vi "Get Page VI.vi"(8 "error in (no error)":errorcluster, 9 "GUID":string, 10 "Item Ref":T1 format="%.0x", 11 "System Explorer Dispatcher Implementation in":refnum<class "System Explorer Dispatcher Implementation.lvclass">) -> (0 "error out":errorcluster, 2 "page reference":refnum<vi>, 3 "System Explorer Dispatcher Implementation out":refnum<class "System Explorer Dispatcher Implementation.lvclass">)   [LabVIEW 2020, in "Communication Bus Template System Explorer.lvlib" / "Implementation.lvlib" / "System Explorer Dispatcher Implementation.lvclass"]
uses:
  System Explorer Dispatcher Implementation.lvclass
  <vilib>/NI VeriStand/Custom Device API/Custom Device Item Ref.ctl
  Scripting/Constants.vi
  System Explorer/Implementation.lvlib
  Scripting/Communication Bus Template Scripting.lvlib
  <vilib>/NI VeriStand/Custom Device API/Custom Device API.lvlib
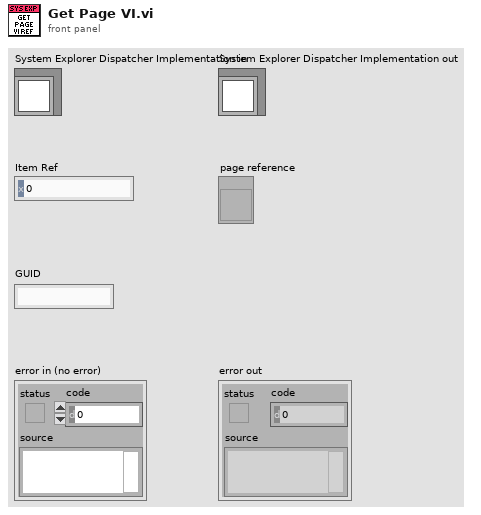
[diagram p1: front panel]
types:
  T1 = typedef "Custom Device API.lvlib/Custom Device Item Ref.ctl" = u64
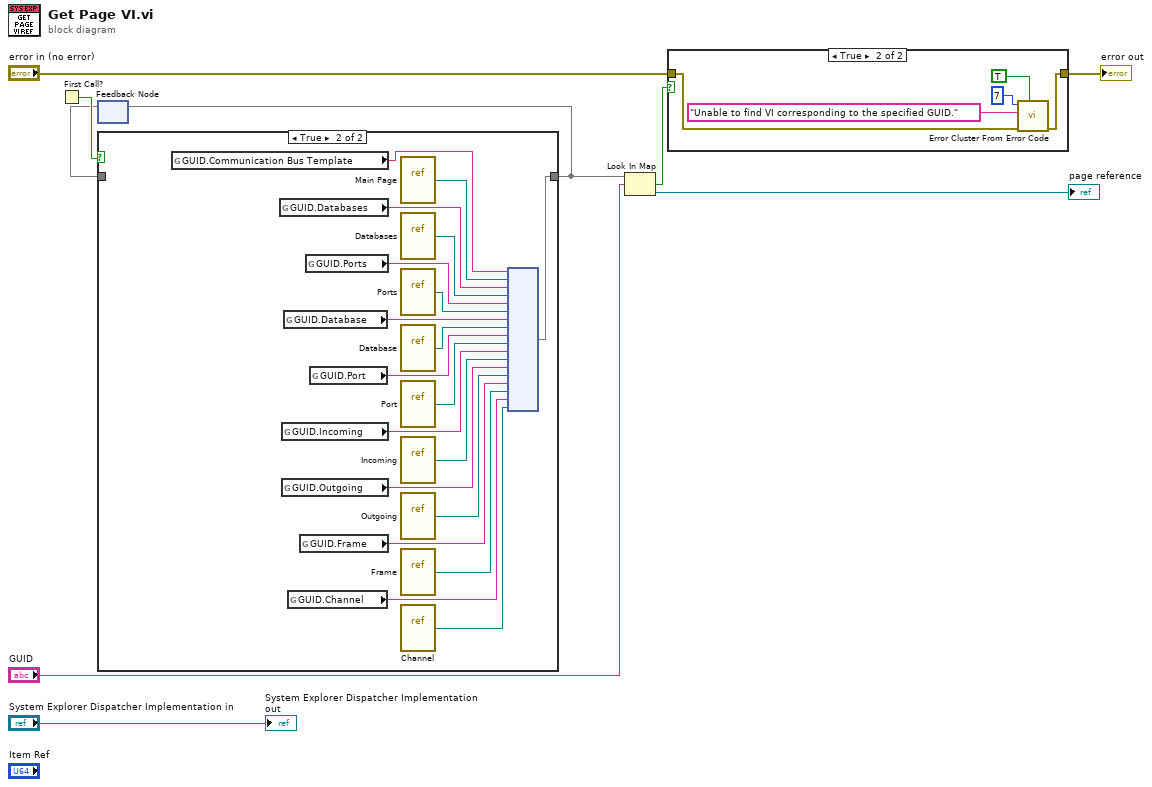
[diagram p0: block diagram]
diagram:
  n1 = First Call?() -> (First Call?: T/F=w8:bool)
  n2 = feedback #1() -> (w7:map{string, refnum<vi>})  [unwired: 1 in]
  n3 = case shown="True" w8 {
    tunnel: [w10 w29] -> w6
    tunnel: w7 -> [w10 _]
    frame False {
    }
    frame True {
      n4 = global read "Constants.vi" "GUID.Communication Bus Template"() -> (w27:string)
      n5 = global read "Constants.vi" "GUID.Databases"() -> (w25:string)
      n6 = global read "Constants.vi" "GUID.Incoming"() -> (w18:string)
      n7 = global read "Constants.vi" "GUID.Outgoing"() -> (w16:string)
      n8 = global read "Constants.vi" "GUID.Database"() -> (w22:string)
      n9 = global read "Constants.vi" "GUID.Channel"() -> (w11:string)
      n10 = global read "Constants.vi" "GUID.Frame"() -> (w14:string)
      n11 = global read "Constants.vi" "GUID.Ports"() -> (w24:string)
      n12 = global read "Constants.vi" "GUID.Port"() -> (w20:string)
      n13 = vi-ref "Main Page.vi"() -> (w28:refnum<vi>)
      n14 = vi-ref "Databases.vi"() -> (w26:refnum<vi>)
      n15 = vi-ref "Ports.vi"() -> (w23:refnum<vi>)
      n16 = vi-ref "Database.vi"() -> (w21:refnum<vi>)
      n17 = vi-ref "Port.vi"() -> (w19:refnum<vi>)
      n18 = vi-ref "Incoming.vi"() -> (w17:refnum<vi>)
      n19 = vi-ref "Outgoing.vi"() -> (w15:refnum<vi>)
      n20 = vi-ref "Frame.vi"() -> (w13:refnum<vi>)
      n21 = vi-ref "Channel.vi"() -> (w12:refnum<vi>)
      n22 = node(w27, w28, w25, w26, w24, w23, w22, w21, w20, w19, w18, w17, w16, w15, w14, w13, w11, w12) -> (w29:map{string, refnum<vi>})
    }
  }
  n23 = feedback-in #1(w6) -> ()
  n24 = Look In Map(map=w6, key="GUID") -> (key not found?=w4:bool, value=→"page reference":refnum<vi>)  [unwired: 1 in]
  n25 = case shown="True" w4 {
    tunnel: [w30 w32] -> w3
    tunnel: "error in (no error)" -> [w30 w31]
    frame False {
    }
    frame True {
      n26 = call <vilib>:"Error Cluster From Error Code.vi"("show call chain? (False)"=TRUE, "error in (no error)"=w31, "error message (\"\")"="Unable to find VI corresponding to the specified GUID." ("error message (\"\")"), "error code (0)"=7) -> ("error out"=w32:errorcluster)  [unwired: 5 in]
    }
  }
  "error out" <- w3
  "System Explorer Dispatcher Implementation out" <- "System Explorer Dispatcher Implementation in"
